vi "DIO Loop.vi"(9 "DIO value in":bool, 10 "enable output":bool, 11 "DIO line":refnum<k21>="Port0/DIO0") -> (1 "DIO value out":bool)   [LabVIEW 2017, in "NI_Robotics_Starter Kit FPGA.lvlib"]
uses:
  <vilib>/robotics/Starter Kit/FPGA Source/NI_Robotics_Starter Kit FPGA.lvlib
  <vilib>/eio/EIOMethodNode/EIOMethodNode.xnode
  <vilib>/eio/EIONode/EIONode.xnode
  <vilib>/rvi/eio/common/nirviEmuTemplateMethod_errors.vi
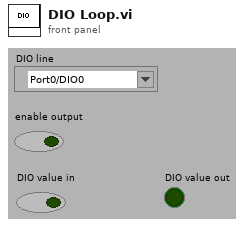
[diagram p1: front panel]
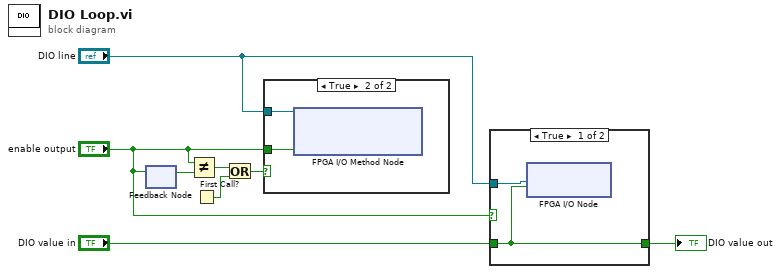
[diagram p0: block diagram]
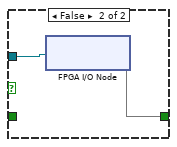
[diagram p2: hidden frame]
diagram:
  n1 = feedback-in #1("enable output") -> ()
  n2 = feedback #1() -> (w8:bool)  [unwired: 1 in]
  n3 = Not Equal?(x="enable output", y=w8) -> (x != y?=w7:bool)
  n4 = First Call?() -> (First Call?: T/F=w6:bool)
  n5 = Or(x=w7, y=w6) -> (x .or. y?=w5:bool)
  n6 = case shown="True" w5 {
    tunnel: "DIO line" -> [_ w10]
    tunnel: "enable output" -> [_ w9]
    frame False {
    }
    frame True {
      n7 = xnode "FPGA I/O Method Node"("FPGA I/O In"=w10, "Enable"=w9) -> ()  [unwired: 1 out]
    }
  }
  n8 = case shown="True" "enable output" {
    tunnel: "DIO line" -> [w12 w14]
    tunnel: "DIO value in" -> [w11 _]
    tunnel: [w11 w13] -> w2
    frame True {
      n9 = xnode "FPGA I/O Node"("I/O Item"=w11, "FPGA I/O In"=w12) -> ()  [unwired: 1 out]
    }
    frame False {
      n10 = xnode "FPGA I/O Node"("FPGA I/O In"=w14) -> ("I/O Item"=w13)  [unwired: 1 out]
    }
  }
  "DIO value out" <- w2
